vi "Safe Angle.vi"(6 "error in (no error)":errorcluster, 7 "Angle":dbl) -> (2 "error out":errorcluster, 3 "Safe Angle":dbl)   [LabVIEW 2015]
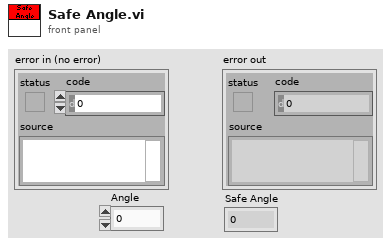
[diagram p1: front panel]
types:
  T1 = typedef "WPI_DigitalInputDevRef.ctl" = cluster{"DevStatus":errorcluster, "DIO Channel":T2}
  T2 = typedef "FPGA_DIOChannel.ctl" = enum8{"DIO 0", "DIO 1", "DIO 2", "DIO 3", "DIO 4", "DIO 5", "DIO 6", "DIO 7", "DIO 8", "DIO 9", "DIO MXP 0", "DIO MXP 1", "DIO MXP 2", "DIO MXP 3", "DIO MXP 4", "DIO MXP 5", "DIO MXP 6", "DIO MXP 7", "DIO MXP 8", "DIO MXP 9", "DIO MXP 10", "DIO MXP 11", "DIO MXP 12", "DIO MXP 13", "DIO MXP 14", "DIO MXP 15", "Invalid"}
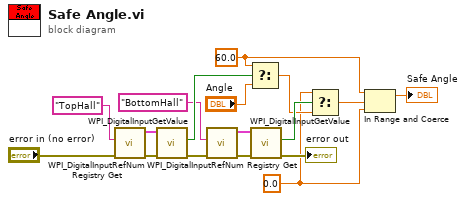
[diagram p0: block diagram]
diagram:
  w3 = 60.0 ("t")
  w2 = 0.0 ("t")
  n1 = call <vilib>:"WPI_DigitalInputRefNum Registry Get.vi"("error in (no error)"="error in (no error)", "refnum name"="TopHall") -> ("error out"=w9:errorcluster, "DigitalInputDevRef"=w10:T1)  [unwired: 8 in]
  n2 = call <vilib>:"WPI_DigitalInputGetValue.vi"("error in (no error)"=w9, "DigitalInputDevRef"=w10) -> ("error out"=w8:errorcluster, "Value"=w16:bool)  [unwired: 7 in, 1 out]
  n3 = call <vilib>:"WPI_DigitalInputRefNum Registry Get.vi"("error in (no error)"=w8, "refnum name"="BottomHall") -> ("error out"=w12:errorcluster, "DigitalInputDevRef"=w11:T1)  [unwired: 8 in]
  n4 = Select(t=w3, s=w16, f="Angle") -> (s? t:f=w5:dbl)
  n5 = call <vilib>:"WPI_DigitalInputGetValue.vi"("error in (no error)"=w12, "DigitalInputDevRef"=w11) -> ("error out"=→"error out":errorcluster, "Value"=w17:bool)  [unwired: 7 in, 1 out]
  n6 = Select(t=w2, s=w17, f=w5) -> (s? t:f=w4:dbl)
  n7 = In Range and Coerce(upper limit=w3, x=w4, lower limit=w2) -> (coerced(x)=→"Safe Angle":dbl)  [unwired: 1 out]
